vi "PB_Cburn_ESR_modified.vi"(5 "# freq points":i32=61, 7 "# scans before track":i32=50, 11 "ESR Modified Parameters":T1={"Window 1 time (s)"=0.012, "Window 2 time (s)"=5e-06, "Window 3 time (s) "=0.02, "Window 4 time (s)"=5e-07, "Window 4 channels"=[TRUE, FALSE, FALSE, TRUE], "Window 3 channels"=[TRUE, FALSE, TRUE, TRUE], "Window 2 channels"=[TRUE, FALSE, FALSE, TRUE], "Window 1 channels"=[TRUE, TRUE, FALSE, TRUE], "Path to ESR Burner"=path "C:/Users/Loncar/Desktop/ESR VIs - Srujan/Sam Kim - ESR remove outliers/PB/ESR_modified_burn.exe", "Window 5 time (s)"=1.0, "Drive channel"=5} {"Drive channel" max=8}) -> ()   [LabVIEW 2012]
uses:
  ESR Modified Window Parameters.ctl
panel:
  out "String":string
  # "MW freq step\ndwell time"
  # "MW freq step"
  # "Wait"
  # "Fluorescence\ncounting"
  # "Ctr sample clk"
  # "Wait"
  # "Wait between\nfreq sweeps"
  # "On/off between freq sweeps (off first)"
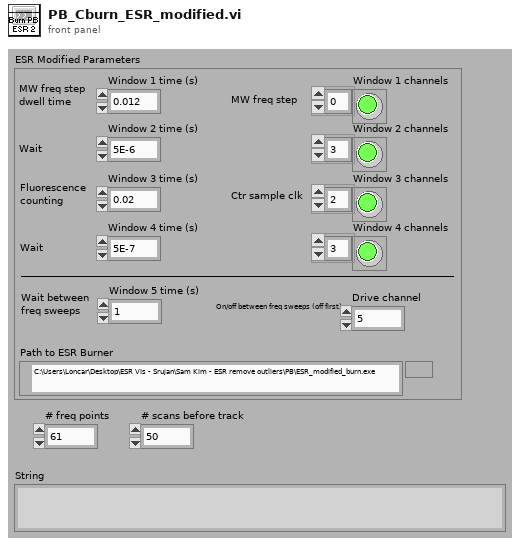
[diagram p1: front panel]
types:
  T1 = typedef "ESR Modified Window Parameters.ctl" = cluster{"Window 1 time (s)":dbl, "Window 2 time (s)":dbl, "Window 3 time (s) ":dbl, "Window 4 time (s)":dbl, "Window 4 channels":bool[], "Window 3 channels":bool[], "Window 2 channels":bool[], "Window 1 channels":bool[], "Path to ESR Burner":path, "Window 5 time (s)":dbl, "Drive channel":u8}
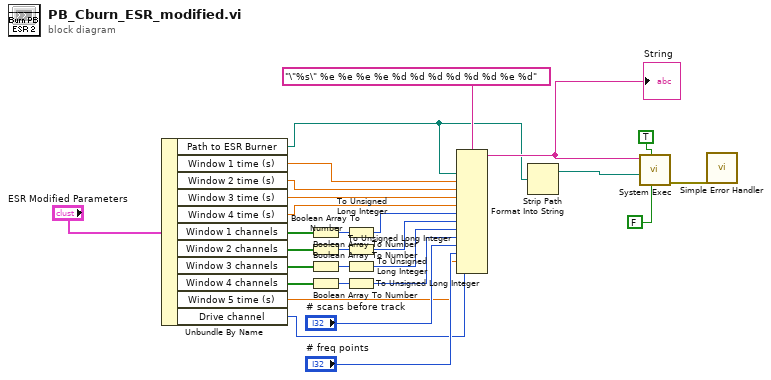
[diagram p0: block diagram]
diagram:
  n1 = Unbundle By Name("ESR Modified Parameters") -> ("Path to ESR Burner"=w4:path, "Window 1 time (s)"=w12:dbl, "Window 2 time (s)"=w11:dbl, "Window 3 time (s)"=w10:dbl, "Window 4 time (s)"=w9:dbl, "Window 1 channels"=w8:bool[], "Window 2 channels"=w7:bool[], "Window 3 channels"=w6:bool[], "Window 4 channels"=w5:bool[], "Window 5 time (s)"=w2:dbl, "Drive channel"=w1:u8)
  n2 = Boolean Array To Number(Boolean array=w8) -> (number=w25:u32)
  n3 = Boolean Array To Number(Boolean array=w7) -> (number=w24:u32)
  n4 = Boolean Array To Number(Boolean array=w6) -> (number=w23:u32)
  n5 = Boolean Array To Number(Boolean array=w5) -> (number=w22:u32)
  n6 = To Unsigned Long Integer(number=w25) -> (unsigned 32bit integer=w21:u32)
  n7 = To Unsigned Long Integer(number=w24) -> (unsigned 32bit integer=w20:u32)
  n8 = To Unsigned Long Integer(number=w23) -> (unsigned 32bit integer=w19:u32)
  n9 = To Unsigned Long Integer(number=w22) -> (unsigned 32bit integer=w18:u32)
  n10 = Format Into String(format string="\"%s\" %e %e %e %e %d %d %d %d %d %d %e %d", w4, w12, w11, w10, w9, w21, w20, w19, w18, "# scans before track", "# freq points", w2, w1) -> (resulting string=w14:string)  [unwired: 2 in, 1 out]
  "String" <- w14
  n11 = Strip Path(path=w4) -> (stripped path=w28:path)  [unwired: 1 out]
  n12 = call <vilib>:"System Exec.vi"("run minimized? (F)"=FALSE ("Wait until done"), "wait until completion? (T)"=TRUE ("Wait until done"), "working directory"=w28, "command line"=w14) -> ("error out"=w13:errorcluster)  [unwired: 4 in, 3 out]
  n13 = call <vilib>:"Simple Error Handler.vi"("error in (no error)"=w13) -> ()  [unwired: 4 in, 5 out]
